vi "숫자형.vi"() -> ()   [LabVIEW 2020]
panel:
  out "결과":dbl
  in  "D":dbl
  in  "C":i32
  in  "B":dbl
  in  "A":dbl
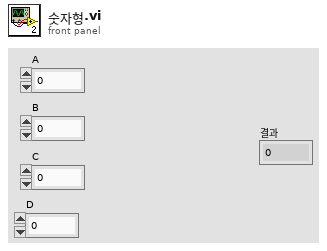
[diagram p1: front panel]
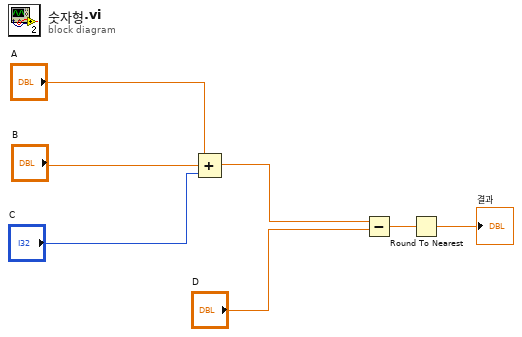
[diagram p0: block diagram]
diagram:
  n1 = Compound Arithmetic op=ADD("A", "B", "C") -> (w4:dbl)
  n2 = Subtract(x=w4, y="D") -> (x-y=w2:dbl)
  n3 = Round To Nearest(number=w2) -> (nearest integer value=→"결과":dbl)
